vi "Acquisition_encodeur.vi"() -> ()   [LabVIEW 2018]
uses:
  <vilib>/Instr/_visa.llb/VISA Configure Serial Port (Instr).vi
panel:
  in  "Tab Control":enum32{"Page 1", "Page 2"}(tab)
  out "Waveform Chart":dynamicdata(graph)
  in  "Consigne":dbl(knob) scale=-360.0..360.0
  out "Mesure":dbl(knob) scale=0.0..360.0
  in  "stop":bool
  in  "VISA resource name":refnum<visa-resource-name>
  # "UNIVESITE SULTAN MOULAY SLIMANE\nFACULTE DES SCIENCES ET TECHNIQUES DE BENI MELLAL"
  # "Réalisé par : BANANE Mohamed\n               IDRRISI Hamza\n                      BELAISSAOUI ARBI\n                          TACHTIOUINE Hicham\n              CHAMIT Salim"
  # "Encadré par : Pr. KHAOUCH Zakaria"
  # "Placez tout \nd'abord le \npendule dans \nsa position d'equilibre \nverticale !"
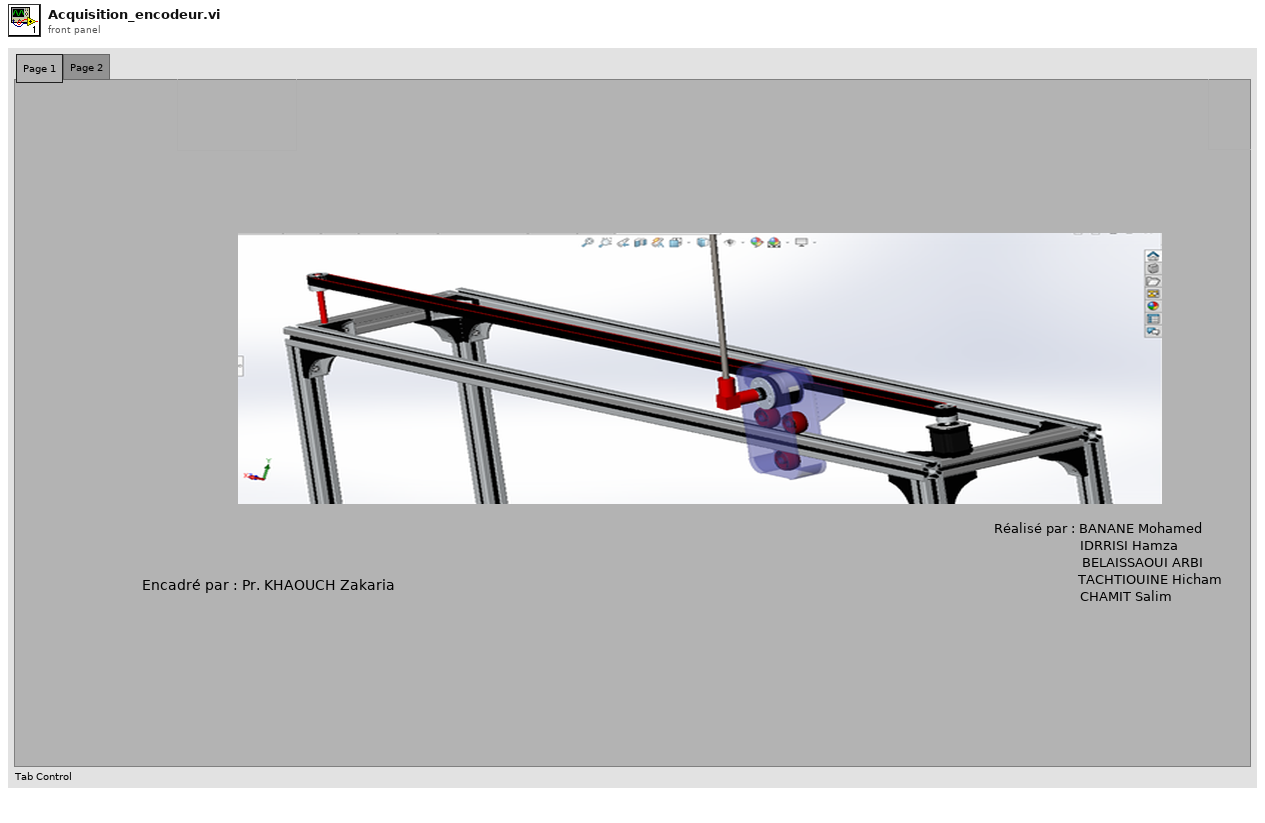
[diagram p1: front panel]
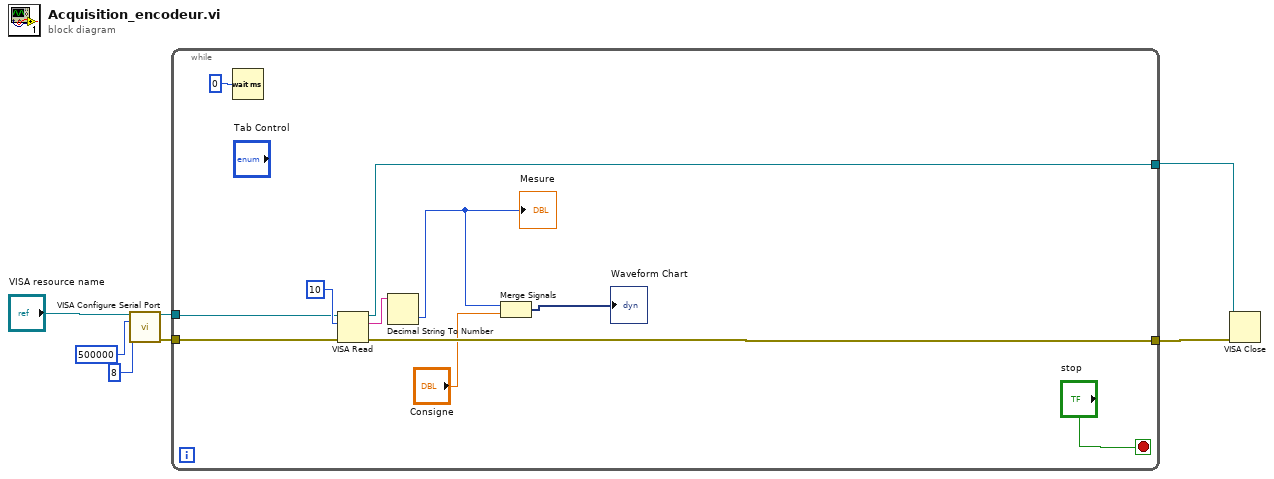
[diagram p0: block diagram]
diagram:
  n1 = call-poly "VISA Configure Serial Port"("VISA resource name"="VISA resource name", "baud rate (9600)"=u32 500000, "data bits (8)"=u16 8) -> ("VISA resource name out"=w3:refnum<visa-resource-name>, "error out"=w2:errorcluster)  [unwired: 11 in]
  n2 = while {
    tunnel: [w15] -> w4
    tunnel: [w14] -> w5
    tunnel: w3 -> [w11]
    tunnel: w2 -> [w10]
    stop <- "stop" stop-if-true
    n3 = Wait (ms)(milliseconds to wait=u32 0) -> ()  [unwired: 1 out]
    n4 = VISA Read(VISA resource name=w11, byte count=u32 10, error in (no error)=w10) -> (VISA resource name out=w15:refnum<visa-resource-name>, read buffer=w16:string, error out=w14:errorcluster)  [unwired: 1 out]
    n5 = Decimal String To Number(string=w16) -> (number=w9:i32)  [unwired: 2 in, 1 out]
    "Mesure" <- w9
    n6 = Merge Signals(w9, "Consigne") -> (→"Waveform Chart":dynamicdata)
  }
  n7 = VISA Close(VISA resource name=w4, error in (no error)=w5) -> ()  [unwired: 1 out]
